vi "CANOpen_Main_Compare RPDO Data for Change.vi"(9 "PDO Settings":T1={"Parameters"=[], "PDO Channel"=1, "Start Index"=0, "Length"=0} {"PDO Channel" items=["PDO 1", "PDO 2", "PDO 3", "PDO 4"]; "Parameters"."Bit Offset" max=8 step=1; "Parameters"."Byte Offset" max=8 step=1}, 10 "Previous Data":dbl[](array[numeric]), 11 "Current Data":dbl[](array[numeric])) -> (2 "Changed?":bool, 3 "Data":dbl[](array[numeric]))   [LabVIEW 2021, in "CANOpen Addon Engine.lvlib"]
uses:
  Shared/CANOpen_PDO Settings.ctl
  Shared/CANOpen_PDO Parameter Settings.ctl
  Shared/CANOpen_PDO Data Type.ctl
  System Explorer/SubVIs/CANopen Byte Order.ctl
  CANOpen Addon Engine.lvlib
  Shared/CANOpen Addon Shared.lvlib
  System Explorer/CANOpen Addon System Explorer.lvlib
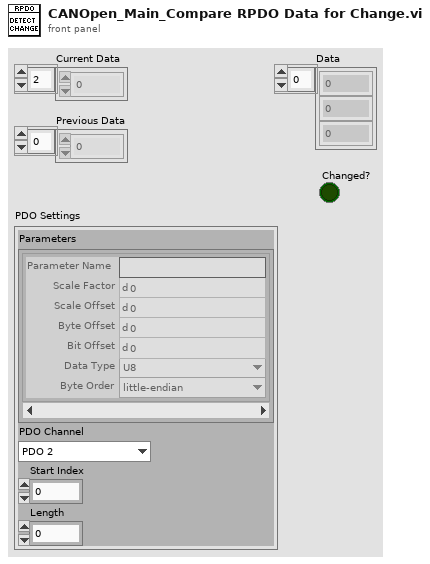
[diagram p1: front panel]
types:
  T1 = typedef "CANOpen Addon Shared.lvlib/CANOpen_PDO Settings.ctl" = cluster{"Parameters":T2[], "PDO Channel":u8, "Start Index":u32, "Length":u32}
  T2 = typedef "CANOpen Addon Shared.lvlib/CANOpen_PDO Parameter Settings.ctl" = cluster{"Parameter Name":string, "Scale Factor":dbl, "Scale Offset":dbl, "Byte Offset":u8, "Bit Offset":u8, "Data Type":T3, "Byte Order":T4}
  T3 = typedef "CANOpen Addon Shared.lvlib/CANOpen_PDO Data Type.ctl" = enum16{"U8", "U16", "U32", "I8", "I16", "I32", "Single", "Double", "Boolean"}
  T4 = typedef "CANOpen Addon System Explorer.lvlib/CANopen Byte Order.ctl" = enum16{"big-endian network order", "little-endian"}
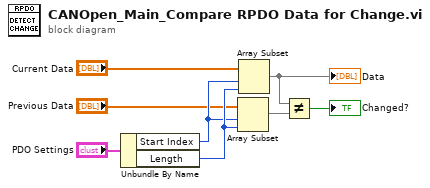
[diagram p0: block diagram]
diagram:
  n1 = Unbundle By Name("PDO Settings") -> ("Start Index"=w4:u32, "Length"=w5:u32)
  n2 = Array Subset(array="Previous Data", index=w4, length=w5) -> (w6:dbl[])
  n3 = Array Subset(array="Current Data", index=w4, length=w5) -> (w8:dbl[])
  "Data" <- w8
  n4 = Not Equal?(x=w8, y=w6) -> (x != y?=→"Changed?":bool)
